vi "GlobalVariables.vi"() -> ()   [LabVIEW 2018, in "Keithley 2600 Series.lvlib"]
uses:
  Keithley 2600 Series.lvlib
panel:
  in  "Error Query":bool=TRUE
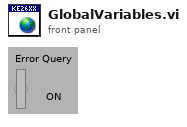
[diagram p1: front panel]
diagram:
